vi "Choreo_Util_AllianceFlipTranslation3d.vi"(11 "Translation":T1 {"Z" format="%14.3f"; "Y" format="%14.3f"; "X" format="%14.3f"}) -> (3 "FlippedTranslation":T1 {"Z" format="%14.3f"; "Y" format="%14.3f"; "X" format="%14.3f"})   [LabVIEW 2019, in "ChoreoLib.lvlib"]
doc: "Flips a translation3d cluster.\n\nInputs: \n -- translation - translation3d - The translation to flip.\n\nOutputs:\n -- FlippedTranslation - Translation3d - The flipped cluster"
uses:
  ChoreoLib.lvlib
  <vilib>/Rock Robotics/WPI/ThirdParty/JAS_Junk/TrajLib/TypeDef/TRANSLATION3D.ctl
  Choreo_Choreo_Globals.vi
  <vilib>/Rock Robotics/WPI/ThirdParty/JAS_Junk/TrajLib/Trajectory_Library.lvlib
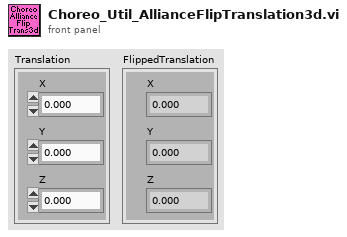
[diagram p1: front panel]
types:
  T1 = typedef "Trajectory_Library.lvlib/TRANSLATION3D.ctl" = cluster{"X":dbl, "Y":dbl, "Z":dbl}
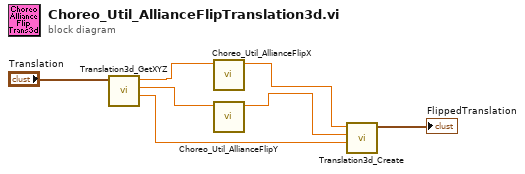
[diagram p0: block diagram]
diagram:
  n1 = call <vilib>:"Translation3d_GetXYZ.vi"("In Translation3d"="Translation") -> ("Z"=w1:dbl, "Y"=w2:dbl, "X"=w3:dbl)  [unwired: 8 in]
  n2 = call "Choreo_Util_AllianceFlipX.vi"("X"=w3) -> ("FlippedX"=w5:dbl)  [unwired: 10 in]
  n3 = call "Choreo_Util_AllianceFlipY.vi"("Y"=w2) -> ("FlippedY"=w4:dbl)  [unwired: 10 in]
  n4 = call <vilib>:"Translation3d_Create.vi"("Z"=w1, "Y"=w4, "X"=w5) -> ("TRANSLATION3D"=→"FlippedTranslation":T1)  [unwired: 8 in]
